vi "define.vi"(8 "error in (no error)":errorcluster, 11 "TrajectoryDL110413StraightLine in":refnum<class "TrajectoryDL110413StraightLine.lvclass">) -> (0 "error out":errorcluster, 3 "TrajectoryDL110413StraightLine out":refnum<class "TrajectoryDL110413StraightLine.lvclass">)   [LabVIEW 2010, in "TrajectoryDL110413StraightLine.lvclass"]
doc: "modal dialog on which the user can set the trajectory parameters"
uses:
  TrajectoryDL110413StraightLine.lvclass
  common/xcontrols/XImage/XImage/XImage.xctl
  common/classes/ImageCollection/ImageCollection/ImageCollection.lvclass
  TrajectoryDL110413StraightLine.lvclass/TrajectoryDL110413StraightLine.ctl
panel:
  in  "cancelButton":bool
  in  "okButton":bool
  in  "Tab Control":enum32{"User", "About"}(tab)
  in  "bidirectional?":bool
  in  "number of pixels":i32
  in  "XImage":refnum<class "ImageCollection.lvclass">(xcontrol)
  # "TrajectoryDL110413StraightLine\n\nimplemented by: Dominik Langer, University of Zurich, Switzerland"
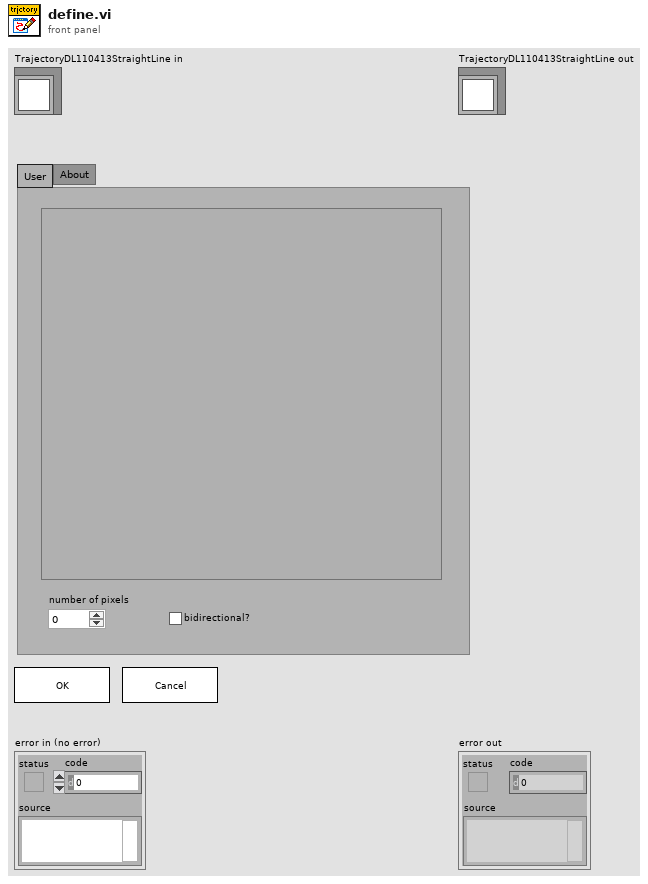
[diagram p1: front panel]
types:
  T1 = typedef "ROImicrons_frames_cluster.ctl" = cluster{"ROI":cluster{"Global Rectangle":dbl[unit][], "Contours":cluster{"Contour Type":u32, "ROI Type":u32, "Points":dbl[unit][]}[]}[]}
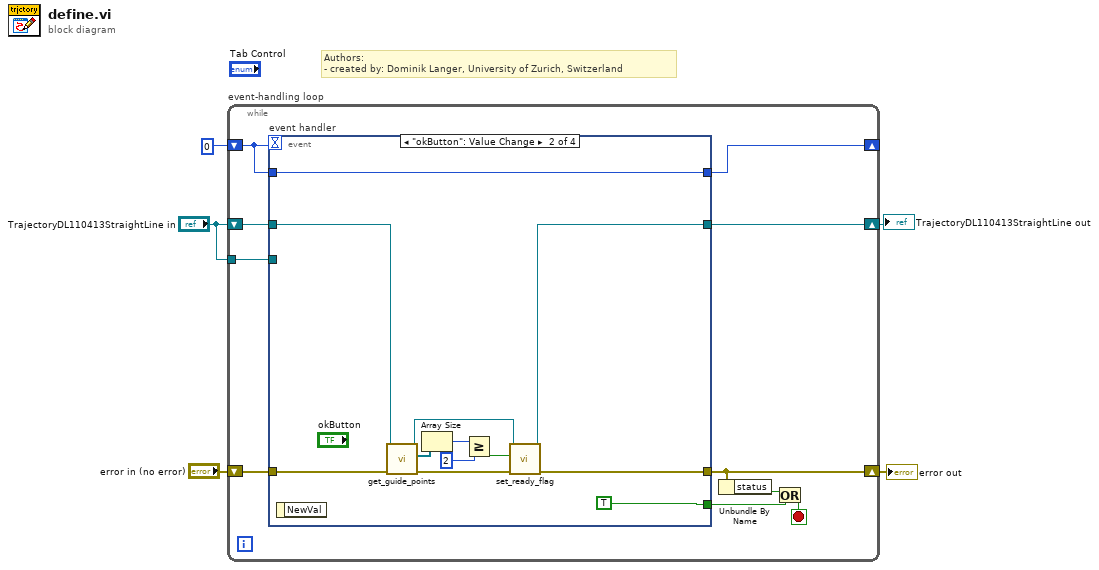
[diagram p0: block diagram]
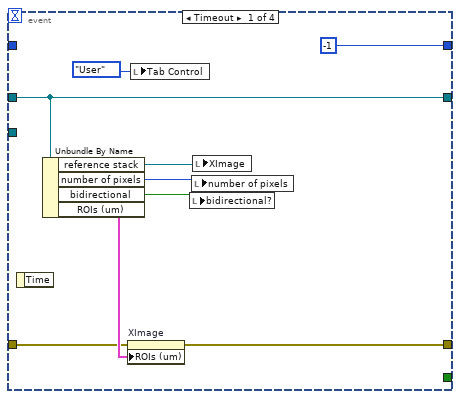
[diagram p2: hidden frame]
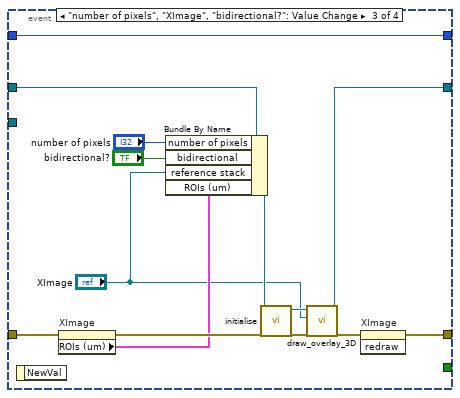
[diagram p3: hidden frame]
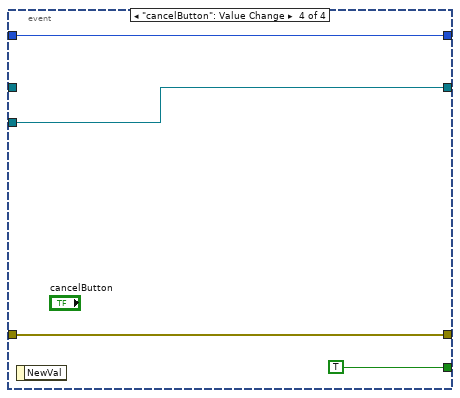
[diagram p4: hidden frame]
diagram:
  # "Authors: \n- created by: Dominik Langer, University of Zurich, Switzerland"
  n1 = while "event-handling loop" {
    shift-right: [w13] -> w4
    shift-left: "error in (no error)" -> [w15]
    shift-right: [w8] -> _
    shift-left: 0 -> [w9]
    shift-right: [w6] -> w3
    shift-left: "TrajectoryDL110413StraightLine in" -> [w14]
    tunnel: "TrajectoryDL110413StraightLine in" -> [w7]
    stop <- w10 stop-if-true
    n2 = event "event handler" shown="[1] \"okButton\": Value Change" {
      selector: _ -> [_ _ _ _]
      dyn-events: _ -> [_ _ _ _]
      timeout: w9 -> [_ _ _ _]
      tunnel: [w18 w34 w38 w54] -> w13
      tunnel: w15 -> [w19 w29 w43 w54]
      tunnel: w14 -> [w22 w26 w48 _]
      tunnel: [w22 w33 w44 w51] -> w6
      tunnel: [_ TRUE _ TRUE] -> w11
      tunnel: [-1 w35 w50 w52] -> w8
      tunnel: w9 -> [_ w35 w50 w52]
      tunnel: w7 -> [_ _ _ w51]
      event Timeout {
        n3 = event-data() -> ()  [unwired: 1 in, 1 out]
        n4 = Unbundle By Name(w22) -> ("reference stack"=w21:refnum<class "ImageCollection.lvclass">, "number of pixels"=w17:i32, "bidirectional"=w16:bool, "ROIs (um)"=w20:T1)
        n5 = property on="XImage" class="XImage (strict)"(error in=w19, "ROIs (um)"=w20) -> (error out=w18:errorcluster)  [unwired: 1 in, 1 out]
        n6 = local write "Tab Control"(enum32{"User", "About"}."User" ("Tab Control")) -> ()
        n7 = local write "bidirectional?"(w16) -> ()
        n8 = local write "number of pixels"(w17) -> ()
        n9 = local write "XImage"(w21) -> ()
      }
      event "okButton": Value Change {
        n10 = event-data() -> ()  [unwired: 1 in, 1 out]
        n11 = call-dynamic "get_guide_points.vi"("error in (no error)"=w29, "TrajectoryDL110413StraightLine in"=w26) -> ("error out"=w28:errorcluster, "guide points"=w27:refnum<class "SpaceVector.lvclass">[], "TrajectoryDL110413StraightLine out"=w25:refnum<class "TrajectoryDL110413StraightLine.lvclass">)  [unwired: 7 in]
        n12 = Array Size(array=w27) -> (size(s)=w32:i32)
        n13 = Greater Or Equal?(x=w32, y=2) -> (x >= y?=w30:bool)
        n14 = call-dynamic "set_ready_flag.vi"("error in (no error)"=w28, "ready for initialisation?"=w30, "GenericTrajectory in"=w25) -> ("error out"=w34:errorcluster, "GenericTrajectory out"=w33:refnum<class "TrajectoryDL110413StraightLine.lvclass">)  [unwired: 7 in]
      }
      event "number of pixels", "XImage", "bidirectional?": Value Change {
        n15 = event-data() -> ()  [unwired: 1 in, 1 out]
        n16 = property on="XImage" class="XImage (strict)"(error in=w43) -> (error out=w42:errorcluster, "ROIs (um)"=w41:T1)  [unwired: 1 in, 1 out]
        n17 = Bundle By Name(cluster=w48, "number of pixels"="number of pixels", "bidirectional"="bidirectional?", "reference stack"="XImage", "ROIs (um)"=w41) -> (w47:refnum<class "TrajectoryDL110413StraightLine.lvclass">)
        n18 = call-dynamic "initialise.vi"("error in (no error)"=w42, "GenericTrajectory in"=w47) -> ("error out"=w46:errorcluster, "GenericTrajectory out"=w45:refnum<class "TrajectoryDL110413StraightLine.lvclass">)  [unwired: 8 in]
        n19 = call-dynamic "draw_overlay_3D.vi"("error in (no error)"=w46, "ImageCollection in"="XImage", "GenericTrajectory in"=w45) -> ("error out"=w39:errorcluster, "GenericTrajectory out"=w44:refnum<class "TrajectoryDL110413StraightLine.lvclass">)  [unwired: 6 in, 1 out]
        n20 = invoke on="XImage" class="XImage (strict)" method="redraw"(error in=w39) -> (error out=w38:errorcluster)  [unwired: 2 in, 2 out]
      }
      event "cancelButton": Value Change {
        n21 = event-data() -> ()  [unwired: 1 in, 1 out]
      }
    }
    n22 = Unbundle By Name(w13) -> ("status"=w12:bool)
    n23 = Or(x=w12, y=w11) -> (x .or. y?=w10:bool)
  }
  "error out" <- w4
  "TrajectoryDL110413StraightLine out" <- w3
